vi "SendVarious.vi"(7 "Boolean_In":bool=TRUE, 8 "error in (no error)":errorcluster, 9 "Array_in":i32[](array[numeric]), 10 "Cluster_In":T1, 11 "reference in":refnum<class "PerformanceTest.lvclass">) -> (0 "error out":errorcluster, 1 "Array_Out":i32[](array[numeric]), 2 "Cluster_Out":T1, 3 "reference out":refnum<class "PerformanceTest.lvclass">, 4 "Boolean_Out":bool=TRUE)   [LabVIEW 2018, in "PerformanceTest.lvclass"]
uses:
  PerformanceTest.lvclass
  ComplexData.ctl
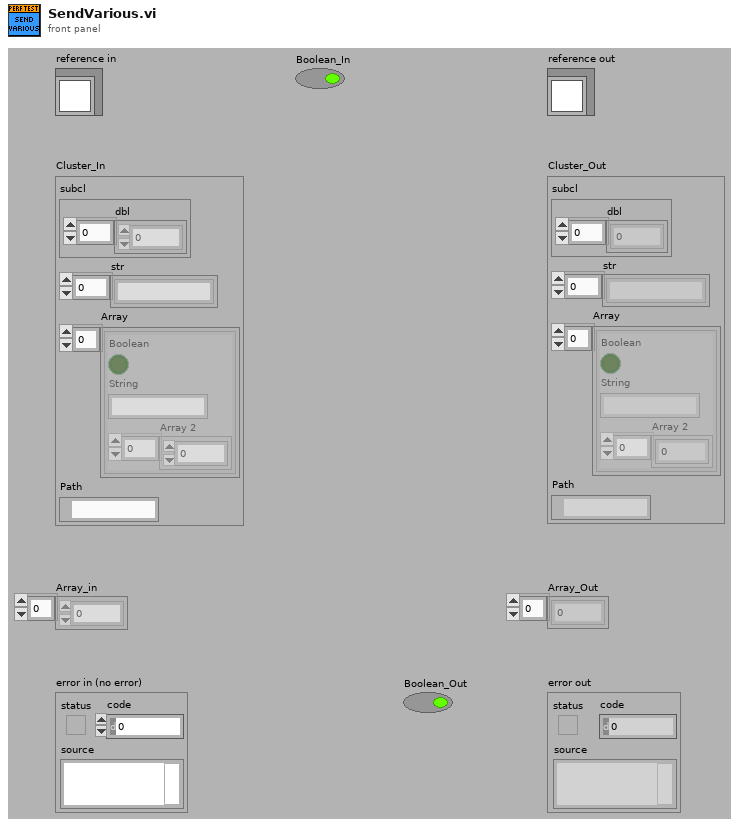
[diagram p1: front panel]
types:
  T1 = typedef "PerformanceTest.lvclass/ComplexData.ctl" = cluster{"subcl":cluster{"dbl":dbl[]}, "str":string[], "Array":cluster{"Boolean":bool, "String":string, "Array 2":dbl[]}[], "Path":path}
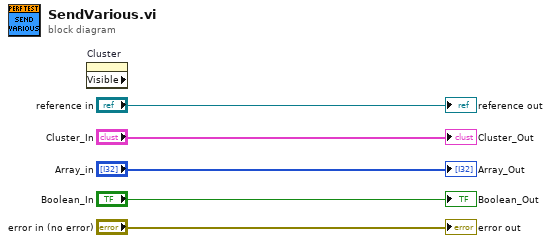
[diagram p0: block diagram]
diagram:
  n1 = property on="Cluster" class="Clust (strict)" props=["Visible"]() -> ()  [unwired: 2 in, 3 out]
  "error out" <- "error in (no error)"
  "reference out" <- "reference in"
  "Cluster_Out" <- "Cluster_In"
  "Array_Out" <- "Array_in"
  "Boolean_Out" <- "Boolean_In"
